vi "set AOI.vi"(8 "error in (no error)":errorcluster, 11 "Thorcam in":refnum<class "Thorcam.lvclass">) -> (0 "error out":errorcluster, 3 "Thorcam out":refnum<class "Thorcam.lvclass">)   [LabVIEW 2012, in "Thorcam.lvclass"]
uses:
  Thorcam.lvclass
  Thorcam.lvclass/Thorcam.ctl
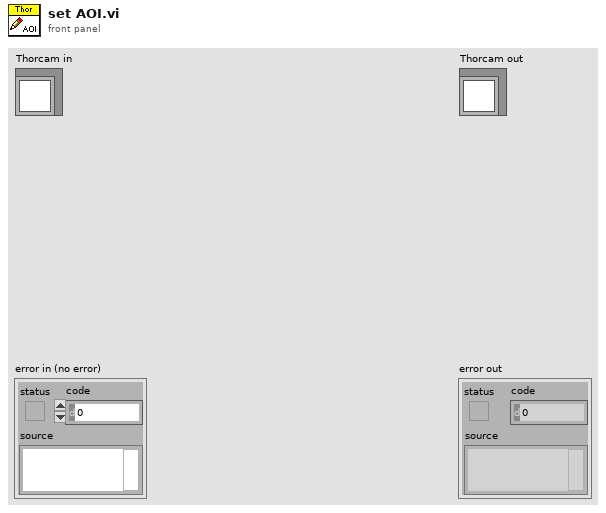
[diagram p1: front panel]
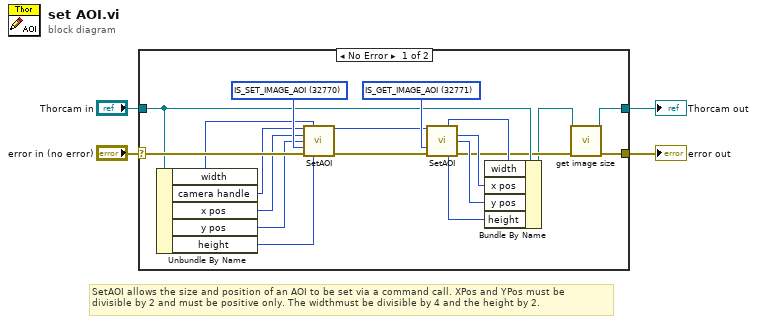
[diagram p0: block diagram]
diagram:
  # "SetAOI allows the size and position of an AOI to be set via a command call. XPos and YPos must be\ndivisible by 2 and must be positive only. The widthmust be divisible by 4 and the height by 2."
  n1 = case shown="No Error" "error in (no error)" {
    selector: "error in (no error)" -> [w23 w25]
    tunnel: [w7 w25] -> w3
    tunnel: [w6 w24] -> w1
    tunnel: "Thorcam in" -> [w9 w24]
    frame No Error {
      w11 = 32771 items=["IS_SET_IMAGE_AOI"=32770, "IS_GET_IMAGE_AOI"=32771] ("Mode")
      w22 = 32770 items=["IS_SET_IMAGE_AOI"=32770, "IS_GET_IMAGE_AOI"=32771] ("Mode")
      n2 = Unbundle By Name(w9) -> ("width"=w21:i32, "camera handle"=w20:u32, "x pos"=w19:i32, "y pos"=w18:i32, "height"=w17:i32)
      n3 = call <instrlib>:"SetAOI.vi"("Camera Handle In"=w20, "Width In"=w21, "XPos In"=w19, "YPos In"=w18, "Mode"=w22, "error in"=w23, "Height In"=w17) -> ("Camera Handle Out"=w10:u32, "error out"=w12:errorcluster)  [unwired: 3 in, 4 out]
      n4 = call <instrlib>:"SetAOI.vi"("Camera Handle In"=w10, "Mode"=w11, "error in"=w12) -> ("Width Out"=w16:i32, "XPos Out"=w14:i32, "YPos Out"=w13:i32, "Height Out"=w15:i32, "error out"=w8:errorcluster)  [unwired: 7 in, 1 out]
      n5 = Bundle By Name(cluster=w9, "width"=w16, "x pos"=w14, "y pos"=w13, "height"=w15) -> (w5:refnum<class "Thorcam.lvclass">)
      n6 = call-dynamic "get image size.vi"("error in (no error)"=w8, "Thorcam in"=w5) -> ("error out"=w7:errorcluster, "Thorcam out"=w6:refnum<class "Thorcam.lvclass">)  [unwired: 6 in, 2 out]
    }
    frame Error {
    }
  }
  "error out" <- w3
  "Thorcam out" <- w1
